vi "PulsePlusOne.vi"(1 "Tree Name":string="proto_tree") -> (0 "Shot #":i32)   [LabVIEW 2013]
uses:
  <vilib>/MDSplus/Library/MDSplus.lvlib
  <vilib>/MDSplus/Classes/Tree_Class/Tree.lvclass
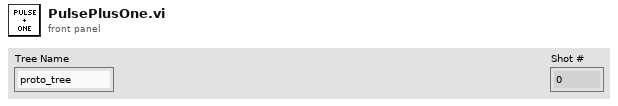
[diagram p1: front panel]
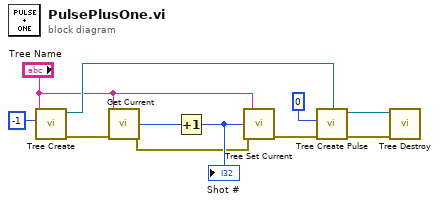
[diagram p0: block diagram]
diagram:
  n1 = call <vilib>:"Tree Create.vi"("Shot"=-1, "Name"="Tree Name") -> ("error out"=w8:errorcluster, "Tree DVR out"=w2:refnum<data-value>)  [unwired: 8 in]
  n2 = call <vilib>:"Get Current.vi"("error in (no error)"=w8, "Tree name"="Tree Name") -> ("error out"=w5:errorcluster, "Current shot out"=w7:i32)  [unwired: 7 in, 1 out]
  n3 = Increment(x=w7) -> (x+1=w6:i32)
  "Shot #" <- w6
  n4 = call <vilib>:"Tree Set Current.vi"("error in (no error)"=w5, "Shot"=w6, "Tree name"="Tree Name") -> ("error out"=w3:errorcluster)  [unwired: 7 in, 1 out]
  n5 = call <vilib>:"Tree Create Pulse.vi"("error in (no error)"=w3, "Shot"=0, "Tree DVR in"=w2) -> ("error out"=w10:errorcluster, "Tree DVR out"=w9:refnum<data-value>)  [unwired: 7 in]
  n6 = call <vilib>:"Tree Destroy.vi"("error in (no error)"=w10, "Tree DVR in"=w9) -> ()  [unwired: 9 in, 1 out]
